vi "Global_SM_Data Out.vi"() -> ()   [LabVIEW 2017, in "Climber.lvlib"]
uses:
  Climber.lvlib
panel:
  out "SM_Climber_VBus":dbl
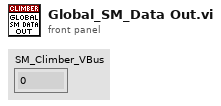
[diagram p1: front panel]
diagram:
